vi "NI VeriStand - Open Command Line Notification (Macro Recorder).vi"(8 "error in (no error)":errorcluster, 11 "MacroRecorder in":T2) -> (0 "error out":errorcluster, 2 "CommandLine Refs":T1, 3 "MacroRecorder out":T2)   [LabVIEW 2020, in "NI_VS MacroRecorderAPI.lvlib"]
doc: "Opens a reference to the command line of the Macro Recorder tool. Opening this reference enables you to use the Get Macro Recorder Command Lines VI to read the commands the VeriStand Gateway sends to the RT target or desktop PC. This VI also returns a user event that you can register and wire to an Event structure."
uses:
  <vilib>/NI VeriStand/Execution/MacroRecorder/NI_VS MacroRecorderAPI.lvlib
  <vilib>/NI VeriStand/Execution/MacroRecorder/MacroRecorderAPI.ctl
  NationalInstruments.VeriStand.ClientAPI
  <vilib>/NI VeriStand/Execution/MacroRecorder/CommandLine Refs.ctl
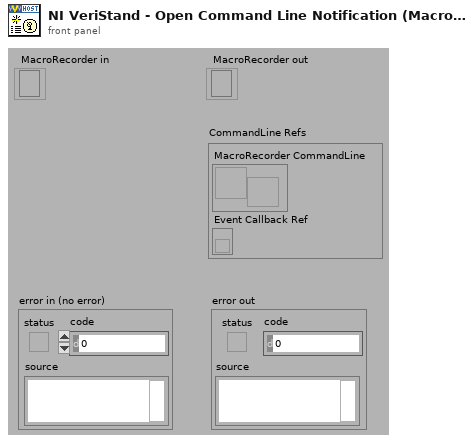
[diagram p1: front panel]
types:
  T1 = typedef "NI_VS MacroRecorderAPI.lvlib/CommandLine Refs.ctl" = cluster{"MacroRecorder CommandLine":refnum<user-event>, "Event Callback Ref":refnum<k27>}
  T2 = typedef "NI_VS MacroRecorderAPI.lvlib/MacroRecorderAPI.ctl" = refnum<k24>
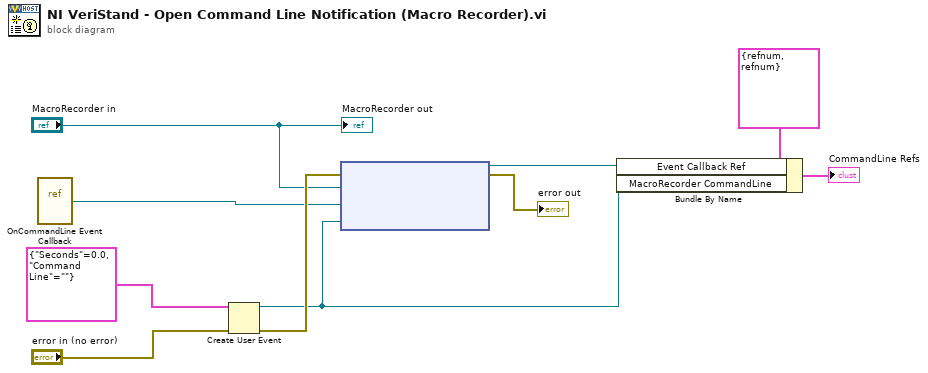
[diagram p0: block diagram]
diagram:
  n1 = vi-ref <vilib>:"OnCommandLine Event Callback.vi"() -> ("vi reference"=w1:refnum<vi>)
  n2 = Create User Event(user event datatype=cluster{"Seconds":dbl, "Command Line":string} {"Seconds"=0.0, "Command Line"=""} ("output cluster"), error in="error in (no error)") -> (user event=w5:refnum<user-event>, error out=w10:errorcluster)
  n3 = node(w10, "MacroRecorder in", w1, w5) -> (w4:refnum<k27>, →"error out":errorcluster)  [unwired: 1 in]
  n4 = Bundle By Name(cluster=T1 {"MacroRecorder CommandLine"=refnum, "Event Callback Ref"=refnum} ("CommandLine Refs"), "Event Callback Ref"=w4, "MacroRecorder CommandLine"=w5) -> (→"CommandLine Refs":T1)
  "MacroRecorder out" <- "MacroRecorder in"
